vi "myPICO_AWG.vi"(11 "数组":T1(array[cluster])) -> ()   [LabVIEW 2024]
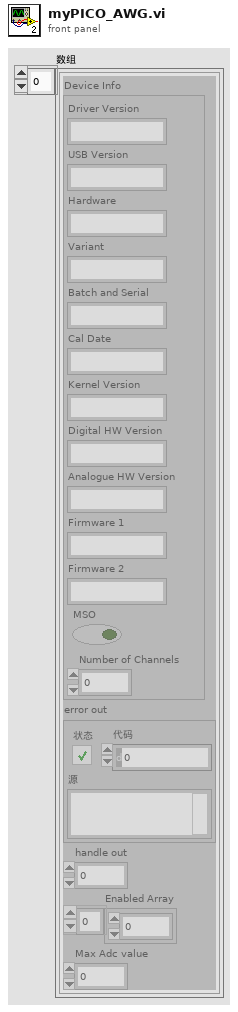
[diagram p1: front panel]
types:
  T1 = cluster{"Device Info":cluster{"Driver Version":string, "USB Version":string, "Hardware":string, "Variant":string, "Batch and Serial":string, "Cal Date":string, "Kernel Version":string, "Digital HW Version":string, "Analogue HW Version":string, "Firmware 1":string, "Firmware 2":string, "MSO":bool, "Number of Channels":i16}, "error out":errorcluster, "handle out":i16, "Enabled Array":i16[], "Max Adc value":i16}[]
  T2 = cluster{"Peak-to-Peak Voltage (microvolts)":u32, "Offset Voltage (microvolts)":i32, "Wave Type":i16, "Sweep Type":i32, "Shots":u32, "Sweeps":u32, "Trigger Type":i32, "Trigger Source":i32, "Ext. Threshold (ADC count)":i16, "White Noise":bool}
  T3 = cluster{"Arbirary waveform file path":path, "Index Mode":u32}
  T4 = cluster{"Start Frequency":dbl, "Stop Frequency":dbl, "Increment":dbl, "Dwell Time (seconds)":dbl}
  T5 = cluster{"Device Info":cluster{"Driver Version":string, "USB Version":string, "Hardware":string, "Variant":string, "Batch and Serial":string, "Cal Date":string, "Kernel Version":string, "Digital HW Version":string, "Analogue HW Version":string, "Firmware 1":string, "Firmware 2":string, "MSO":bool, "Number of Channels":i16}, "error out":errorcluster, "handle out":i16, "Enabled Array":i16[], "Max Adc value":i16}
  T6 = cluster{"Driver Version":string, "USB Version":string, "Hardware":string, "Variant":string, "Batch and Serial":string, "Cal Date":string, "Kernel Version":string, "Digital HW Version":string, "Analogue HW Version":string, "Firmware 1":string, "Firmware 2":string, "MSO":bool, "Number of Channels":i16}
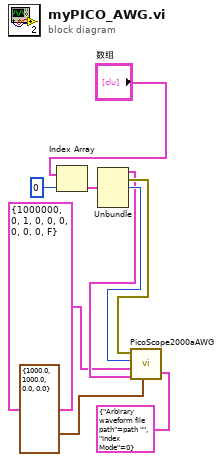
[diagram p0: block diagram]
diagram:
  n1 = Index Array(array="数组", index=0 ("索引")) -> (element=w5:T5)
  n2 = Unbundle(w5) -> ("Device Info"=w7:T6, "error out"=w8:errorcluster, "handle out"=w9:i16)  [unwired: 2 out]
  n3 = call "PicoScope2000aAWG.vi"("Arbitrary Waveform Settings"=T3 {"Arbirary waveform file path"=path "", "Index Mode"=0}, "Standard Waveform Settings"=T4 {"Start Frequency"=1000.0, "Stop Frequency"=1000.0, "Increment"=0.0, "Dwell Time (seconds)"=0.0}, "Device Info"=w7, "General AWG Settings"=T2 {"Peak-to-Peak Voltage (microvolts)"=1000000, "Offset Voltage (microvolts)"=0, "Wave Type"=1, "Sweep Type"=0, "Shots"=0, "Sweeps"=0, "Trigger Type"=0, "Trigger Source"=0, "Ext. Threshold (ADC count)"=0, "White Noise"=FALSE} ("General AWG Settings 2"), "Handle In"=w9, "error in"=w8) -> ()  [unwired: 2 in, 4 out]
